vi "Kikusui PLZ-Read Measurements.vi"(8 "error in":errorcluster, 11 "Kikusui PLZ Setting In":T1={"VISA Resource Name"="", "Baud Rate"=19200, "Stop Bits"=20, "Wait For Read(ms)"=0} {"Stop Bits" items=["1.0"=10, "2.0"=20]; "Baud Rate" items=["2400"=2400, "4800"=4800, "9600"=9600, "19200"=19200]}) -> (0 "error out":errorcluster, 2 "Measurement Data":T2, 3 "Kikusui PLZ Setting Out":T1={"VISA Resource Name"="", "Baud Rate"=19200, "Stop Bits"=20, "Wait For Read(ms)"=0} {"Stop Bits" items=["1.0"=10, "2.0"=20]; "Baud Rate" items=["2400"=2400, "4800"=4800, "9600"=9600, "19200"=19200]})   [LabVIEW 2018]
uses:
  Data Def/Kikusui PLZ-Measurement Data.ctl
  Data Def/Kikusui PLZ-Setting.ctl
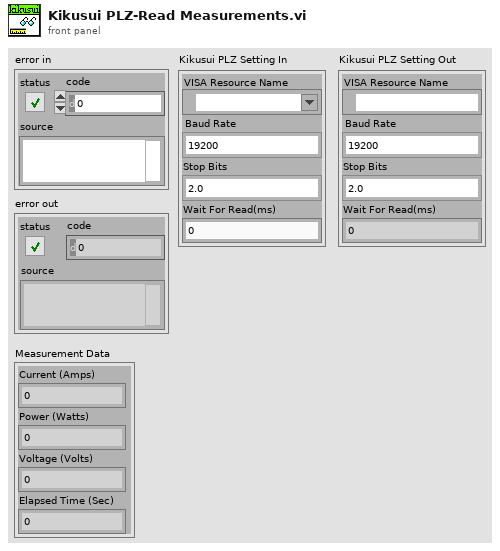
[diagram p1: front panel]
types:
  T1 = typedef "Kikusui PLZ-Setting.ctl" = cluster{"VISA Resource Name":refnum<visa-resource-name>, "Baud Rate":u32, "Stop Bits":u16, "Wait For Read(ms)":u32}
  T2 = typedef "Kikusui PLZ-Measurement Data.ctl" = cluster{"Current (Amps)":dbl, "Power (Watts)":dbl, "Voltage (Volts)":dbl, "Elapsed Time (Sec) ":dbl}
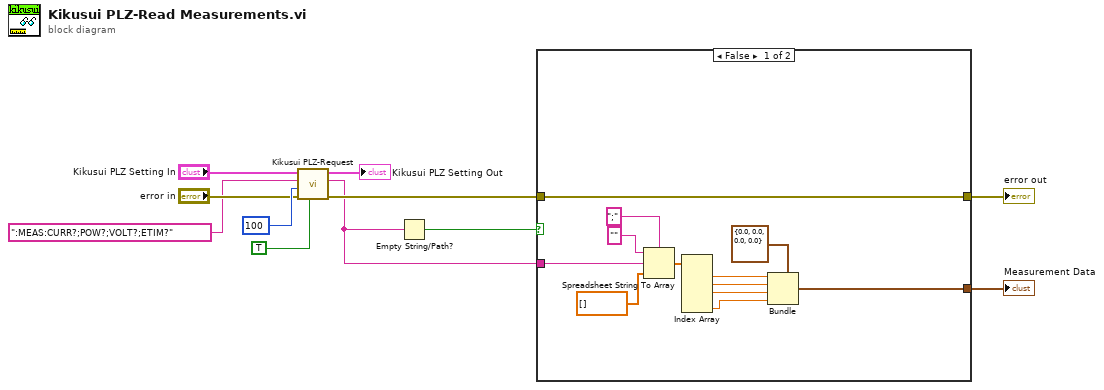
[diagram p0: block diagram]
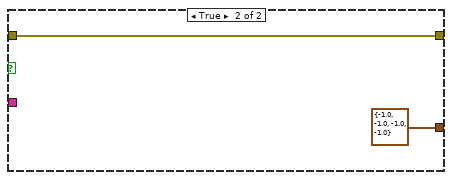
[diagram p2: hidden frame]
diagram:
  n1 = call "Kikusui PLZ-Request.vi"("Response?"=TRUE, "error in"="error in", "byte count"=u32 100, "Command"=":MEAS:CURR?;POW?;VOLT?;ETIM?" ("Current,Power,Voltage and Elapsed Time Measurement Command"), "Kikusui PLZ Setting In"="Kikusui PLZ Setting In") -> ("error out"=w11:errorcluster, "Response"=w7:string, "Kikusui PLZ Setting Out"=→"Kikusui PLZ Setting Out":T1)  [unwired: 4 in]
  n2 = Empty String/Path?(string/path=w7) -> (empty?=w8:bool)
  n3 = case shown="False" w8 {
    tunnel: w11 -> [w17 w25]
    tunnel: [w17 w25] -> w10
    tunnel: [w22 T2 {"Current (Amps)"=-1.0, "Power (Watts)"=-1.0, "Voltage (Volts)"=-1.0, "Elapsed Time (Sec) "=-1.0} ("Measurement Data")] -> w9
    tunnel: w7 -> [w19 _]
    frame False {
      n4 = Spreadsheet String To Array(delimiter (Tab)=";", format string="", spreadsheet string=w19, array type (2D Dbl)=dbl[] []) -> (array=w16:dbl[])
      n5 = Index Array(array=w16) -> (element #1=w15:dbl, element #2=w14:dbl, element #3=w13:dbl, element #5=w12:dbl)  [unwired: 5 in, 1 out]
      n6 = Bundle(cluster=T2 {"Current (Amps)"=0.0, "Power (Watts)"=0.0, "Voltage (Volts)"=0.0, "Elapsed Time (Sec) "=0.0} ("Measurement Data"), "Current (Amps)"=w15, "Power (Watts)"=w14, "Voltage (Volts)"=w13, "Elapsed Time (Sec)"=w12) -> (w22:T2)
    }
    frame True {
    }
  }
  "error out" <- w10
  "Measurement Data" <- w9
